vi "GV stage triggers acquisition.vi"() -> ()   [LabVIEW 2017]
panel:
  out "StageTrigAcq":bool
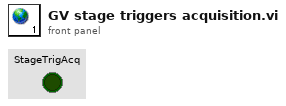
[diagram p1: front panel]
diagram:
